vi "ATS_ErrorDisplay.vi"(5 "error IN":errorcluster) -> (1 "End Out":bool)   [LabVIEW 2015]
doc: "_____AlazarTech, Scope_____\n\nDisplay the error value.\n\nEnd: output set to TRUE\nContinue: End set to False."
panel:
  in  "ABORT":bool
  in  "End":bool
  in  "Continue":bool
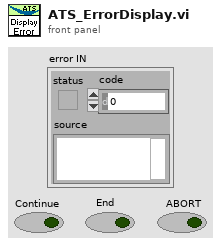
[diagram p1: front panel]
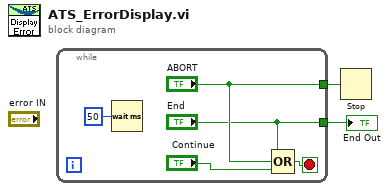
[diagram p0: block diagram]
diagram:
  n1 = while {
    tunnel: ["End"] -> w2
    tunnel: ["ABORT"] -> w1
    stop <- w6 stop-if-true
    n2 = Wait (ms)(milliseconds to wait=u32 50) -> ()  [unwired: 1 out]
    n3 = Compound Arithmetic op=OR("End", "ABORT", "Continue") -> (w6:bool)
  }
  "End Out" <- w2
  n4 = Stop(stop? (T)=w1) -> ()
